vi "Determine Entry Clicked.vi"(8 "error in (no error)":errorcluster, 10 "Byte Position":i32, 11 "BreadcrumbNavigation in":refnum<class "BreadcrumbNavigator.lvclass">) -> (0 "error out":errorcluster, 3 "BreadcrumbNavigation out":refnum<class "BreadcrumbNavigator.lvclass">)   [LabVIEW 2015, in "BreadcrumbNavigator.lvclass"]
uses:
  BreadcrumbNavigator.lvclass
  BreadcrumbNavigator.lvclass/BreadcrumbNavigator.ctl
  Read Strings[].vi
  Read CurrentLeftMostItem.vi
  Read Delimeter.vi
  Write Strings[].vi
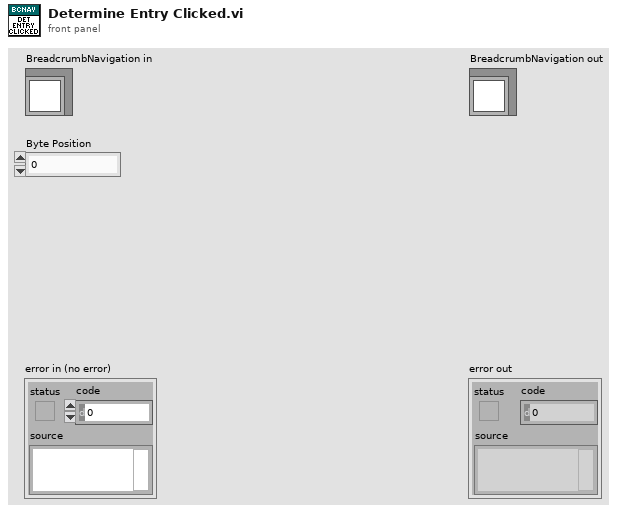
[diagram p1: front panel]
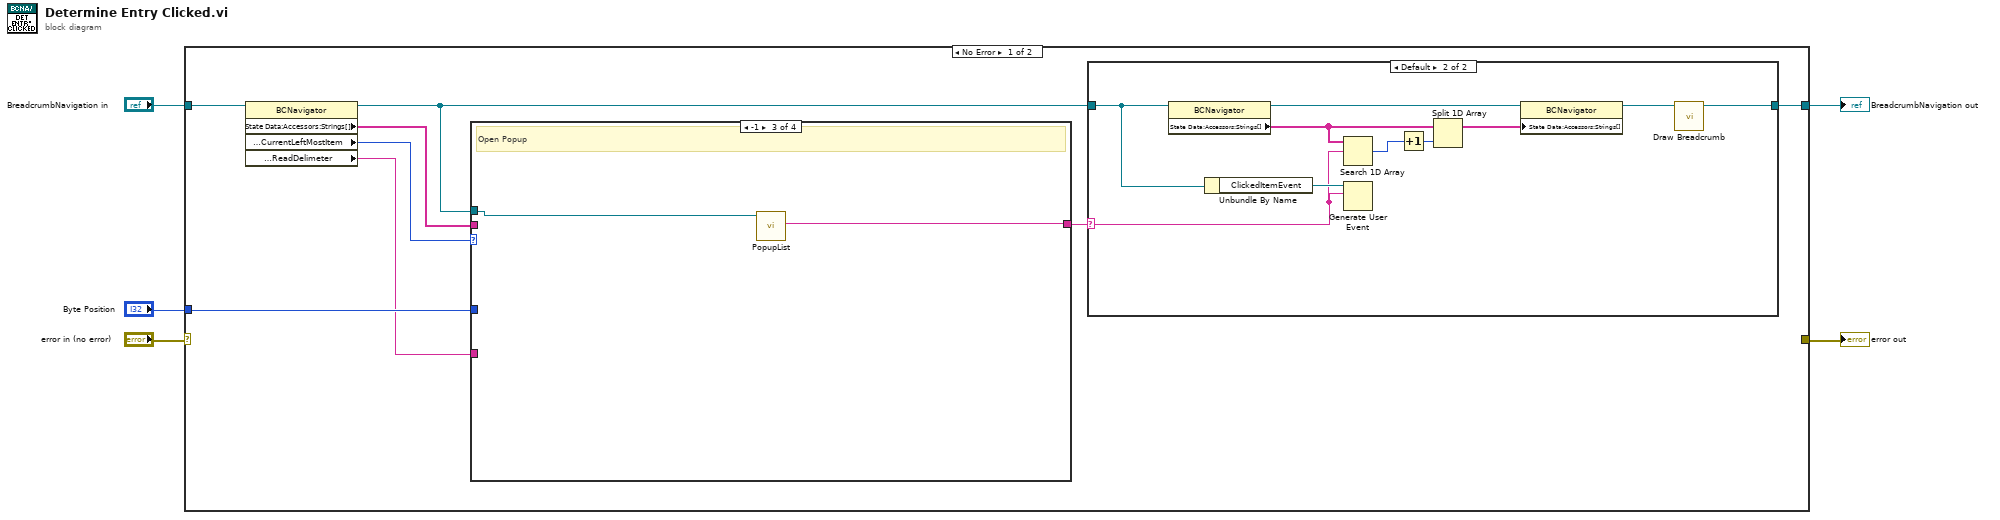
[diagram p0: block diagram]
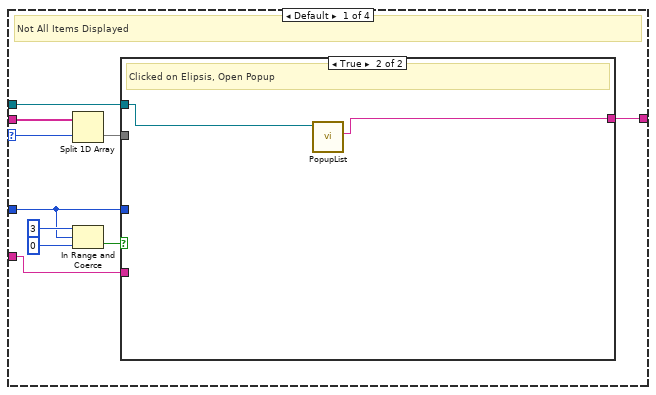
[diagram p3: hidden frame]
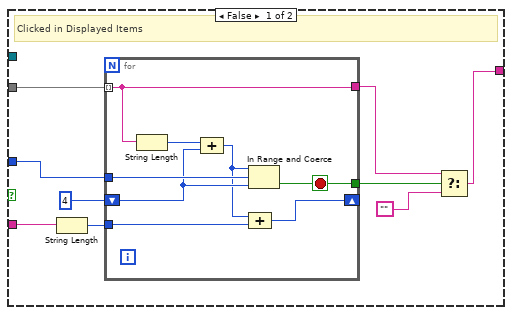
[diagram p4: hidden frame]
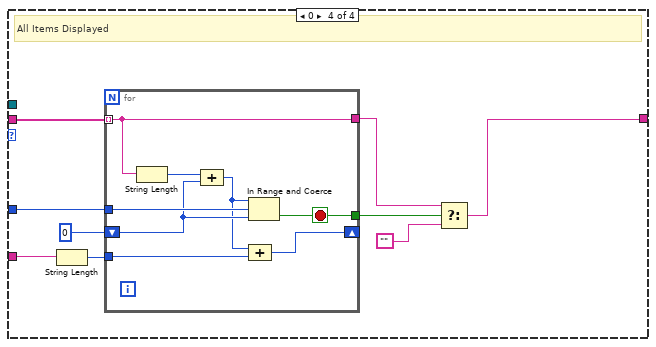
[diagram p6: hidden frame]
diagram:
  n1 = case shown="No Error" "error in (no error)" {
    selector: "error in (no error)" -> [_ w74]
    tunnel: [_ w74] -> w4
    tunnel: [w7 w73] -> w2
    tunnel: "BreadcrumbNavigation in" -> [w13 w73]
    tunnel: "Byte Position" -> [w10 _]
    frame No Error {
      n2 = property class="BCNavigator"(reference=w13) -> (reference out=w6:refnum<class "BreadcrumbNavigator.lvclass">, "State Data:Accessors:Strings[]"=w12:string[], "State Data:Accessors:CurrentLeftMostItem"=w11:i32, "State Data:Accessors:ReadDelimeter"=w9:string)  [unwired: 1 in, 1 out]
      n3 = case shown="-1" w11 {
        selector: w11 -> [w33 _ _ _]
        tunnel: w12 -> [w34 _ _ w63]
        tunnel: w10 -> [w28 _ _ w62]
        tunnel: w9 -> [w27 _ _ w64]
        tunnel: [w26 _ w55 w56] -> w8
        tunnel: w6 -> [w25 _ w54 _]
        frame Default {
          # "Not All Items Displayed"
          n4 = Split 1D Array(array=w34, index=w33) -> (second subarray=w29:string[])  [unwired: 1 out]
          n5 = In Range and Coerce(upper limit=3, x=w28, lower limit=0) -> (In Range?=w30:bool)  [unwired: 1 out]
          n6 = case shown="True" w30 {
            tunnel: w29 -> [w41 _]
            tunnel: w28 -> [w40 _]
            tunnel: w27 -> [w39 _]
            tunnel: [w35 w52] -> w26
            tunnel: w25 -> [_ w53]
            frame False {
              # "Clicked in Displayed Items"
              n7 = String Length(string=w39) -> (length=w43:i32)
              n8 = for {
                tunnel: w41 -> [w48] mode=indexing
                tunnel: w40 -> [w51]
                shift-right: [w49] -> _
                shift-left: 4 -> [w46]
                tunnel: w43 -> [w50]
                tunnel: [w48] -> w36
                tunnel: [w44] -> w37
                stop <- w44 stop-if-true
                n9 = String Length(string=w48) -> (length=w47:i32)
                n10 = Compound Arithmetic op=ADD(w47, w46) -> (w45:i32)
                n11 = In Range and Coerce(upper limit=w45, x=w51, lower limit=w46) -> (In Range?=w44:bool)  [unwired: 1 out]
                n12 = Compound Arithmetic op=ADD(w45, w50) -> (w49:i32)
              }
              n13 = Select(t=w36, s=w37, f="") -> (s? t:f=w35:string)
            }
            frame True {
              # "Clicked on Elipsis, Open Popup"
              n14 = call "PopupList.vi"("BreadcrumbNavigation in"=w53) -> ("SelectedItem"=w52:string)  [unwired: 8 in, 2 out]
            }
          }
        }
        frame -2 {
          # "Array is Empty"
        }
        frame -1 {
          # "Open Popup"
          n15 = call "PopupList.vi"("BreadcrumbNavigation in"=w54) -> ("SelectedItem"=w55:string)  [unwired: 8 in, 2 out]
        }
        frame 0 {
          # "All Items Displayed"
          n16 = String Length(string=w64) -> (length=w60:i32)
          n17 = for {
            tunnel: w63 -> [w69] mode=indexing
            tunnel: w62 -> [w72]
            shift-right: [w70] -> _
            shift-left: 0 -> [w67]
            tunnel: w60 -> [w71]
            tunnel: [w69] -> w57
            tunnel: [w65] -> w59
            stop <- w65 stop-if-true
            n18 = String Length(string=w69) -> (length=w68:i32)
            n19 = Compound Arithmetic op=ADD(w68, w67) -> (w66:i32)
            n20 = In Range and Coerce(upper limit=w66, x=w72, lower limit=w67) -> (In Range?=w65:bool)  [unwired: 1 out]
            n21 = Compound Arithmetic op=ADD(w66, w71) -> (w70:i32)
          }
          n22 = Select(t=w57, s=w59, f="") -> (s? t:f=w56:string)
        }
      }
      n23 = case shown="Default" w8 {
        selector: w8 -> [_ w21]
        tunnel: w6 -> [w14 w24]
        tunnel: [w14 w16] -> w7
        frame "" {
        }
        frame Default {
          n24 = property class="BCNavigator"(reference=w24) -> (reference out=w22:refnum<class "BreadcrumbNavigator.lvclass">, "State Data:Accessors:Strings[]"=w20:string[])  [unwired: 1 in, 1 out]
          n25 = Unbundle By Name(w24) -> ("ClickedItemEvent"=w23:refnum<user-event>)
          n26 = Search 1D Array(1D array=w20, element=w21) -> (index of element=w19:i32)  [unwired: 1 in]
          n27 = Generate User Event(user event=w23, event data cluster=w21) -> ()  [unwired: 2 in, 2 out]
          n28 = Increment(x=w19) -> (x+1=w15:i32)
          n29 = Split 1D Array(array=w20, index=w15) -> (first subarray=w18:string[])  [unwired: 1 out]
          n30 = property class="BCNavigator"(reference=w22, "State Data:Accessors:Strings[]"=w18) -> (reference out=w17:refnum<class "BreadcrumbNavigator.lvclass">)  [unwired: 1 in, 1 out]
          n31 = call "Draw Breadcrumb.vi"("BreadcrumbNavigation in"=w17) -> ("BreadcrumbNavigation out"=w16:refnum<class "BreadcrumbNavigator.lvclass">)  [unwired: 9 in, 1 out]
        }
      }
    }
    frame Error {
    }
  }
  "error out" <- w4
  "BreadcrumbNavigation out" <- w2
